vi "Waveform_Read Write End Point.vi"(7 "Read(f)\nWrite(t)":T1, 10 "End Point":i32, 11 "Raw Data Waveform":T2) -> (2 "Name Out":i32, 3 "Raw Data Waveform Out":T2)   [LabVIEW 2025, in "WavBuf.lvclass"]
uses:
  WavBuf/WavBuf.lvclass
  Universal Controls/Waveform_Data.ctl
  Universal Controls/Read Write Button.ctl
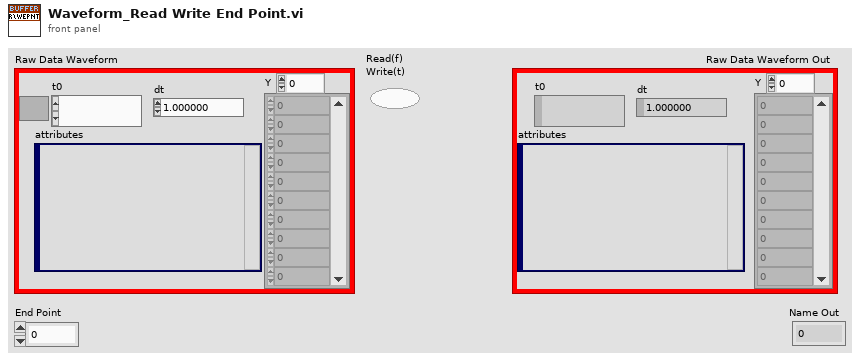
[diagram p1: front panel]
types:
  T1 = typedef "Read Write Button.ctl" = bool
  T2 = typedef "Waveform_Data.ctl" = waveform(dbl)
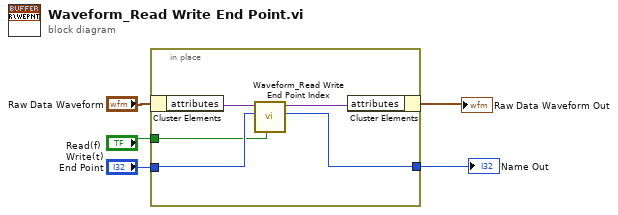
[diagram p0: block diagram]
diagram:
  n1 = in-place {
    in-place-border: "End Point" -> [w8]
    in-place-border: "Read(f)\nWrite(t)" -> [w7]
    in-place-border: [w6] -> w1
    n2 = in-place-cluster #1("Raw Data Waveform") -> ("attributes"=w10:variant)
    n3 = call "Waveform_Read Write End Point Index.vi"("Read(f)\nWrite(t)"=w7, "End Point"=w8, "Waveform Attributes"=w10) -> ("End Point Out"=w6:i32, "Waveform Attributes Out"=w9:variant)  [unwired: 5 in, 2 out]
    n4 = in-place-cluster #1("attributes"=w9) -> (→"Raw Data Waveform Out":T2)
  }
  "Name Out" <- w1
